vi "SDCP TMC Test.vi"() -> ()   [LabVIEW 2020]
uses:
  Typedefs/SDCP - Serial Port Control - Commands.ctl
panel:
  in  "Request Transfer Mode Status":bool
  out "Block Transfer status":bool
  out "Frame Transfer On Request status":bool
  out "Standard Frame Transfer status":bool
  in  "Stop application":bool
  in  "Send transfer mode command":bool
  in  "Block Transfer":bool
  in  "Frame Transfer On Request":bool
  in  "Standard Frame Transfer":bool
  in  "Baud rate":u32=9600
  in  "VISA resource name":refnum<visa-resource-name>
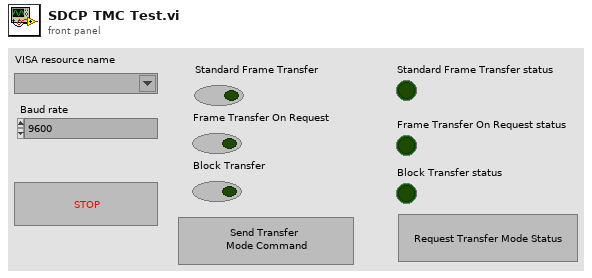
[diagram p1: front panel]
types:
  T1 = typedef "SDCP - Serial Port Control - Commands.ctl" = enum16{"Open", "Read", "Write", "Get instance", "Close"}
  T2 = typedef "SDCP TMC Param.ctl" = cluster{"TMS_REQ":bool, "TMS_ACK":bool, "TMC_REQ":bool, "TMC_ACK":bool, "BTR_ENSTAT":bool, "FTOR_ENSTAT":bool, "SFT_ENSTAT":bool, "BTR_ENREQ":bool, "FTOR_ENREQ":bool, "SFT_ENREQ":bool, "MTR_ENREQ":bool, "MTR_ENACK":bool}
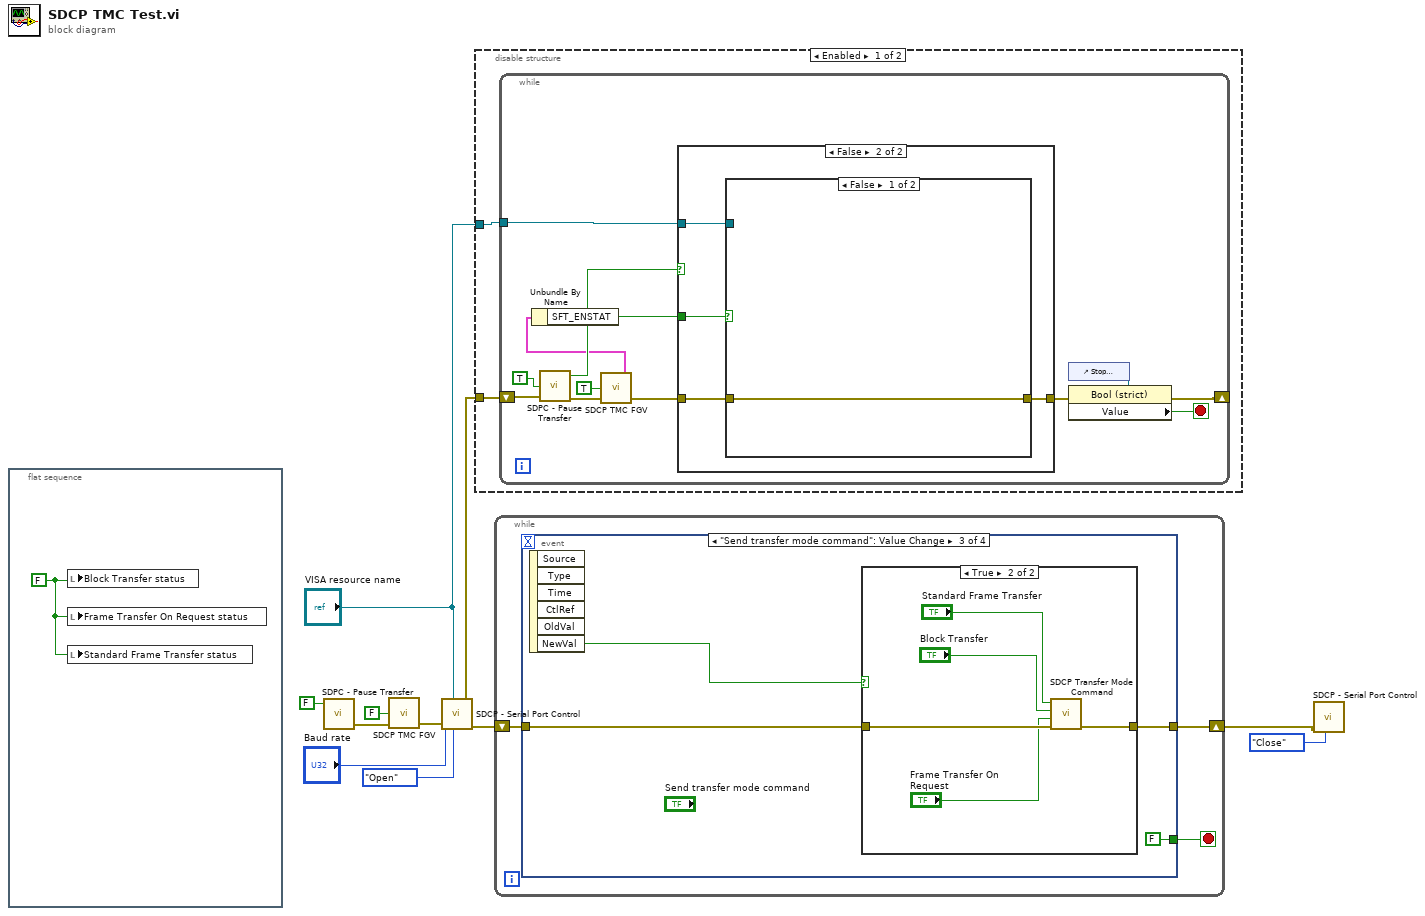
[diagram p0: block diagram]
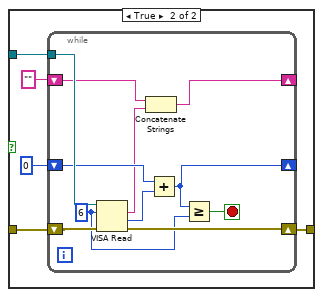
[diagram p3: hidden frame]
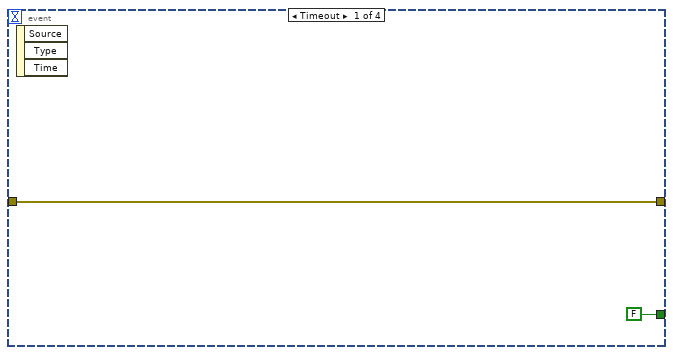
[diagram p5: hidden frame]
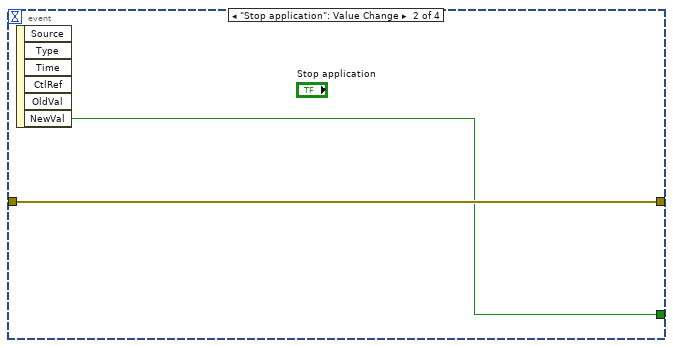
[diagram p6: hidden frame]
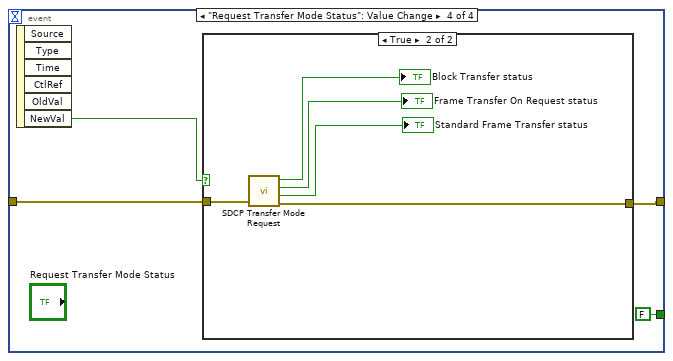
[diagram p8: hidden frame]
diagram:
  n1 = flat-sequence {
    frame #0 {
      w11 = FALSE
      n2 = local write "Block Transfer status"(w11) -> ()
      n3 = local write "Frame Transfer On Request status"(w11) -> ()
      n4 = local write "Standard Frame Transfer status"(w11) -> ()
    }
  }
  n5 = call "SDPC - Pause Transfer.vi"("Pause transfer"=FALSE) -> ("error out"=w2:errorcluster)  [unwired: 3 in, 1 out]
  n6 = call "SDCP TMC FGV.vi"("error in (no error)"=w2, "RD/nWR"=FALSE) -> ("error out"=w6:errorcluster)  [unwired: 2 in, 1 out]
  n7 = call "SDCP - Serial Port Control.vi"("Command"=SDCP_-_Serial_Port_Control_-_Commands."Open", "VISA resource name"="VISA resource name", "error in (no error)"=w6, "Baud rate"="Baud rate") -> ("error out"=w3:errorcluster)  [unwired: 4 in, 3 out]
  n8 = disable-structure shown="Enabled" {
    disable-tunnel: "VISA resource name" -> [w13 _]
    disable-tunnel: w3 -> [w12 _]
    frame Enabled {
      n9 = while {
        shift-right: [w22] -> _
        shift-left: w12 -> [w21]
        tunnel: w13 -> [w24]
        stop <- w25 stop-if-true
        n10 = call "SDPC - Pause Transfer.vi"("error in (no error)"=w21, "RD/nWR"=TRUE) -> ("error out"=w18:errorcluster, "Transfer paused"=w19:bool)  [unwired: 2 in]
        n11 = call "SDCP TMC FGV.vi"("error in (no error)"=w18, "RD/nWR"=TRUE) -> ("error out"=w15:errorcluster, "TMC out"=w16:T2)  [unwired: 2 in]
        n12 = Unbundle By Name(w16) -> ("SFT_ENSTAT"=w14:bool)
        n13 = case shown="False" w19 {
          tunnel: w24 -> [_ w31]
          tunnel: [w27 w30] -> w23
          tunnel: w15 -> [w27 w29]
          tunnel: w14 -> [_ w28]
          frame True {
          }
          frame False {
            n14 = case shown="False" w28 {
              tunnel: w31 -> [_ w37]
              tunnel: [w32 w36] -> w30
              tunnel: w29 -> [w32 w33]
              frame False {
              }
              frame True {
                n15 = while {
                  tunnel: w37 -> [w47]
                  shift-right: [w41] -> w36
                  shift-left: w33 -> [w48]
                  shift-right: [w40] -> _
                  shift-left: 0 -> [w45]
                  shift-right: [w42] -> _
                  shift-left: "" -> [w44]
                  stop <- w38 stop-if-true
                  w39 = u32 6 ("byte count")
                  n16 = VISA Read(VISA resource name=w47, byte count=w39, error in (no error)=w48) -> (read buffer=w43:string, return count=w46:u32, error out=w41:errorcluster)  [unwired: 1 out]
                  n17 = Concatenate Strings(w44, w43) -> (w42:string)
                  n18 = Add(x=w45, y=w46) -> (x+y=w40:u32)
                  n19 = Greater Or Equal?(x=w40, y=w39) -> (x >= y?=w38:bool)
                }
              }
            }
          }
        }
        n20 = control-ref of="Stop application"() -> (w26:refnum<vi>)
        n21 = property class="Bool (strict)"(reference=w26, error in=w23) -> (error out=w22:errorcluster, "Value"=w25:bool)  [unwired: 1 out]
      }
    }
    frame Disabled {
    }
  }
  n22 = while {
    shift-right: [w49] -> w7
    shift-left: w3 -> [w50]
    stop <- w51 stop-if-true
    n23 = event shown="[2] \"Send transfer mode command\": Value Change" {
      selector: _ -> [_ _ _ _]
      dyn-events: _ -> [_ _ _ _]
      timeout: _ -> [_ _ _ _]
      tunnel: [FALSE w54 FALSE ("NewVal") FALSE ("NewVal")] -> w51
      tunnel: w50 -> [w52 w55 w58 w67]
      tunnel: [w52 w55 w56 w66] -> w49
      event Timeout {
        n24 = event-data() -> ()  [unwired: 1 in, 3 out]
      }
      event "Stop application": Value Change {
        n25 = event-data() -> ("NewVal"=w54:bool)  [unwired: 1 in, 5 out]
      }
      event "Send transfer mode command": Value Change {
        n26 = event-data() -> ("NewVal"=w57:bool)  [unwired: 1 in, 5 out]
        n27 = case shown="True" w57 {
          tunnel: w58 -> [w60 w65]
          tunnel: [w60 w64] -> w56
          frame False {
          }
          frame True {
            n28 = call "SDCP Transfer Mode Command.vi"("error in (no error)"=w65, "FTOR"="Frame Transfer On Request", "BTR"="Block Transfer", "SFT"="Standard Frame Transfer") -> ("error out"=w64:errorcluster)  [unwired: 3 in]
          }
        }
      }
      event "Request Transfer Mode Status": Value Change {
        n29 = event-data() -> ("NewVal"=w68:bool)  [unwired: 1 in, 5 out]
        n30 = case shown="True" w68 {
          tunnel: w67 -> [w70 w75]
          tunnel: [w70 w74] -> w66
          frame False {
          }
          frame True {
            n31 = call "SDCP Transfer Mode Request.vi"("error in (no error)"=w75) -> ("BTR"=→"Block Transfer status":bool, "FTOR"=→"Frame Transfer On Request status":bool, "SFT"=→"Standard Frame Transfer status":bool, "error out"=w74:errorcluster)  [unwired: 1 in]
          }
        }
      }
    }
  }
  n32 = call "SDCP - Serial Port Control.vi"("Command"=SDCP_-_Serial_Port_Control_-_Commands."Close", "error in (no error)"=w7) -> ()  [unwired: 6 in, 4 out]
